vi "DpcOpenData.vi"(8 "Error In":errorcluster, 10 "Device Name":string) -> (0 "Error Out":errorcluster, 2 "Task ID":u16, 3 "Device Handle":u32)   [LabVIEW 2011, in "LVH-Adept.lvlib" / "DPCUTIL.lvlib"]
doc: "DPCAPI BOOL DpcOpenData(HANDLE * phif, char * szdvc, ERC * perc, TRID * ptrid);"
uses:
  DPCUTIL.lvlib
  Private/Type Defs/Error.ctl
  <vilib>/LabVIEW Hacker/Adept/Private/Resources/dpcutil.dll
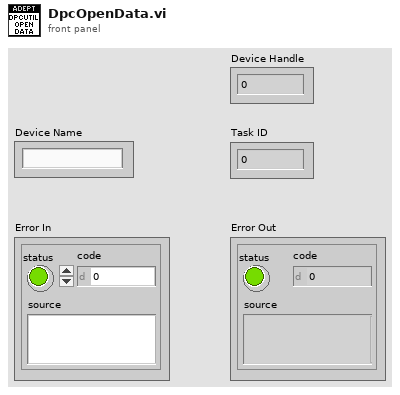
[diagram p1: front panel]
types:
  T1 = typedef "LVH-Adept.lvlib/DPCUTIL.lvlib/Error.ctl" = enum16{"Unknown", "Open Data", "Wait For Transaction", "Put Reg", "Get Reg", "Close Data"}
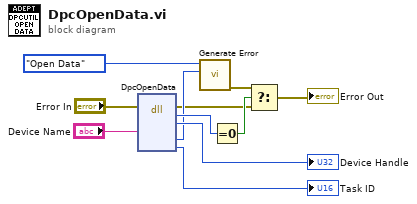
[diagram p0: block diagram]
diagram:
  n1 = dll-call lib="C:/Program Files (x86)/National Instruments/LabVIEW 2011/vi.lib/LabVIEW Hacker/Adept/Private/Resources/dpcutil.*" fn="DpcOpenData"(error in="Error In", "szdvc"="Device Name") -> (error out=w3:errorcluster, "return type"=w8:i32, "phif"=→"Device Handle":u32, "perc"=w5:i32, "ptrid"=→"Task ID":u16)  [unwired: 6 in, 1 out]
  n2 = call "Generate Error.vi"("Adept Error Code"=w5, "DPCUTIL Error"=Error."Open Data") -> ("Error Out"=w6:errorcluster)  [unwired: 9 in]
  n3 = Equal To 0?(x=w8) -> (x = 0?=w9:bool)
  n4 = Select(t=w6, s=w9, f=w3) -> (s? t:f=→"Error Out":errorcluster)
